vi "Load an INI File Listing Other INI Files.vi"(8 "error in (no error)":errorcluster, 11 "configuration file path":path) -> (0 "error out":errorcluster, 3 "Array":path[](array[path]))   [LabVIEW 2017, in "Communications Library.lvlib"]
uses:
  Communications Library.lvlib
  <vilib>/Utility/config.llb/Read Key (Path).vi
  <vilib>/Utility/config.llb/NI_LVConfig.lvlib
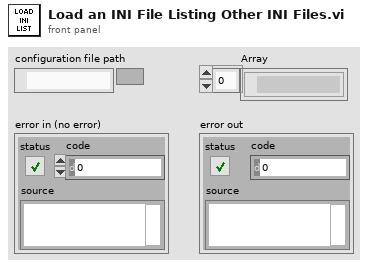
[diagram p1: front panel]
types:
  T1 = typedef "NI_LVConfig.lvlib/Config Data RefNum.ctl" = refnum<k1>
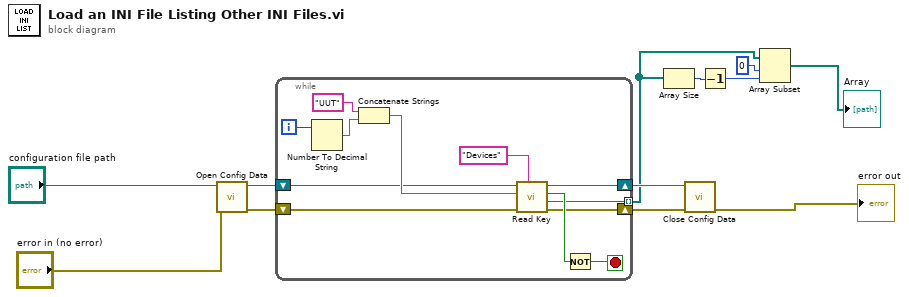
[diagram p0: block diagram]
diagram:
  n1 = call <vilib>:"Open Config Data.vi"("error in (no error)"="error in (no error)", "configuration file path"="configuration file path") -> ("error out"=w7:errorcluster, "refnum"=w10:T1)  [unwired: 7 in, 1 out]
  n2 = while {
    tunnel: [w17] -> w4 mode=indexing
    shift-right: [w15] -> w8
    shift-left: w7 -> [w16]
    shift-right: [w14] -> w9
    shift-left: w10 -> [w13]
    i -> [w23]
    stop <- w19 stop-if-true
    n3 = Number To Decimal String(number=w23) -> (decimal integer string=w21:string)  [unwired: 1 in]
    n4 = Concatenate Strings("UUT" ("section"), w21) -> (w20:string)
    n5 = call-poly <vilib>:"Read Key.vi"("section"="Devices", "error in (no error)"=w16, "key"=w20, "refnum"=w13) -> ("error out"=w15:errorcluster, "value"=w17:path, "found?"=w18:bool, "refnum out"=w14:T1)  [unwired: 4 in]
    n6 = Not(x=w18) -> (.not. x?=w19:bool)
  }
  n7 = Array Size(array=w4) -> (size(s)=w3:i32)
  n8 = call <vilib>:"Close Config Data.vi"("error in (no error)"=w8, "refnum"=w9) -> ("error out"=→"error out":errorcluster)  [unwired: 8 in, 1 out]
  n9 = Decrement(x=w3) -> (x-1=w2:i32)
  n10 = Array Subset(array=w4, index=0, length=w2) -> (→"Array":path[])
